vi "Generate Broken Board.vi"(1 "Assembly Line Input in":refnum<class "Assembly Line Input.lvclass">) -> (0 "Assembly Line Input out":refnum<class "Assembly Line Input.lvclass">)   [LabVIEW 2018, in "Assembly Line Input.lvclass"]
doc: "Generate a board image that will report a test failure in a correctly working system."
uses:
  Assembly Line Input.lvclass
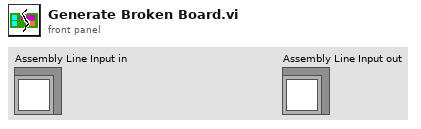
[diagram p1: front panel]
types:
  T1 = cluster{"left":i16, "top":i16, "right":i16, "bottom":i16}
  T2 = typedef "Board Image.ctl" = picture
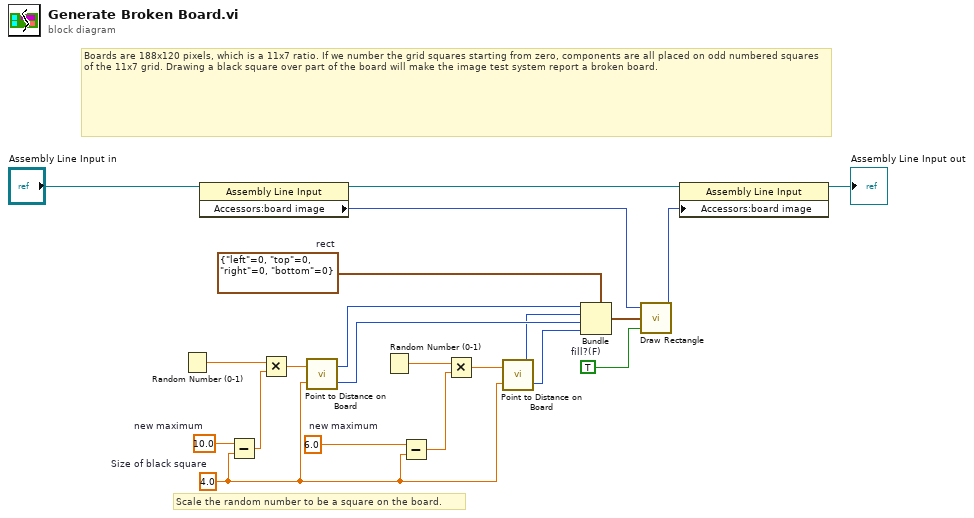
[diagram p0: block diagram]
diagram:
  w11 = 4.0  # Size of black square
  w14 = TRUE  # fill?(F)
  w20 = T1 {"left"=0, "top"=0, "right"=0, "bottom"=0}  # rect
  w13 = 10.0  # new maximum
  w12 = 6.0  # new maximum
  # "Scale the random number to be a square on the board."
  # "Boards are 188x120 pixels, which is a 11x7 ratio. If we number the grid squares starting from zero, components are all placed on odd numbered squares of the 11x7 grid. Drawing a black square over part of the board will make the image test system report a broken board."
  n1 = Random Number (0-1)() -> (number: 0 to 1=w9:dbl)
  n2 = property class="Assembly Line Input"(reference="Assembly Line Input in") -> (reference out=w2:refnum<class "Assembly Line Input.lvclass">, "Accessors:board image"=w4:T2)  [unwired: 1 in, 1 out]
  n3 = Subtract(x=w13, y=w11) -> (x-y=w8:dbl)
  n4 = Multiply(x=w9, y=w8) -> (x*y=w10:dbl)
  n5 = call "Point to Distance on Board.vi"("Size of square"=w11, "scaled value"=w10) -> ("end pixel"=w18:i16, "start pixel"=w19:i16)
  n6 = Random Number (0-1)() -> (number: 0 to 1=w7:dbl)
  n7 = Subtract(x=w12, y=w11) -> (x-y=w5:dbl)
  n8 = Multiply(x=w7, y=w5) -> (x*y=w6:dbl)
  n9 = call "Point to Distance on Board.vi"("Size of square"=w11, "scaled value"=w6) -> ("end pixel"=w16:i16, "start pixel"=w17:i16)
  n10 = Bundle(cluster=w20, "left"=w19, "top"=w17, "right"=w18, "bottom"=w16) -> (w15:T1)
  n11 = call <vilib>:"Draw Rectangle.vi"("picture"=w4, "rect"=w15, "fill?(F)"=w14) -> ("new picture"=w3:picture)  [unwired: 6 in]
  n12 = property class="Assembly Line Input"(reference=w2, "Accessors:board image"=w3) -> (reference out=→"Assembly Line Input out":refnum<class "Assembly Line Input.lvclass">)  [unwired: 1 in, 1 out]
